vi "init_img_processing_vars.vi"(7 "Count Buffer Size 1":i32=2000000) -> (8 "Image Processing Data":T1)   [LabVIEW 2023]
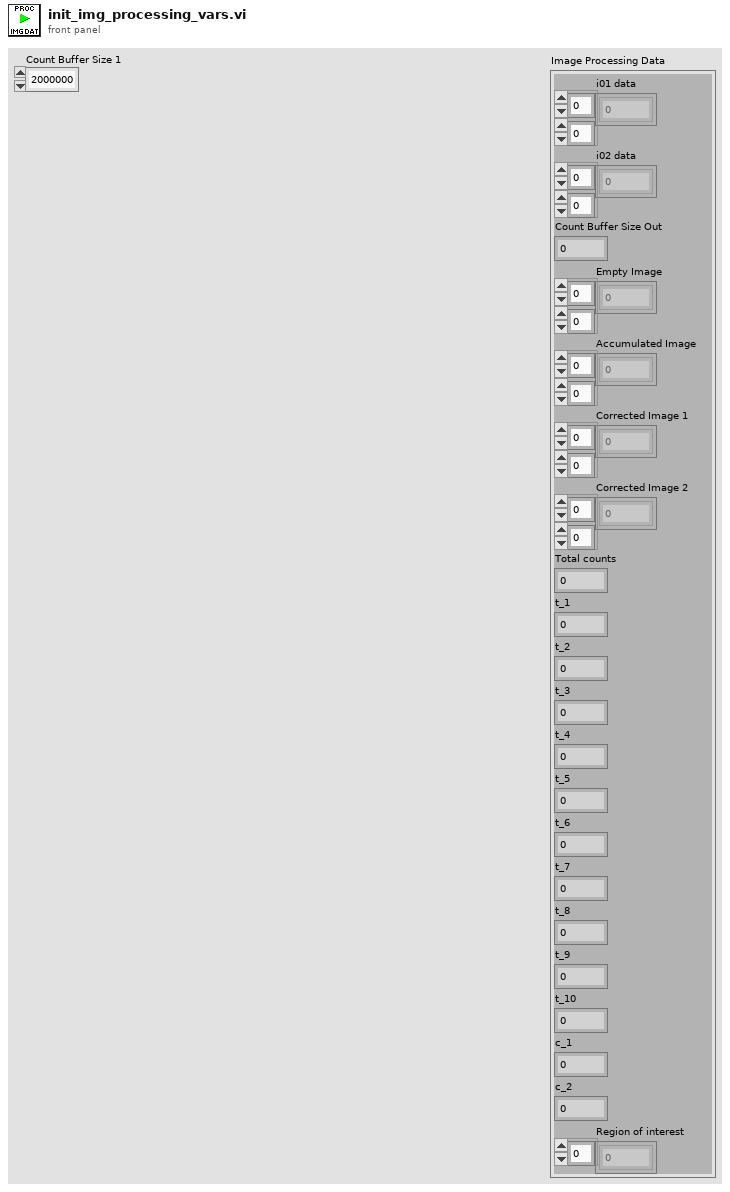
[diagram p1: front panel]
types:
  T1 = cluster{"i01 data":sgl[][], "i02 data":sgl[][], "Count Buffer Size Out":i32, "Empty Image":i16[][], "Accumulated Image":i16[][], "Corrected Image 1":i16[][], "Corrected Image 2":i16[][], "Total counts":i32, "t_1":i32, "t_2":i32, "t_3":i32, "t_4":i32, "t_5":i32, "t_6":i32, "t_7":i32, "t_8":i32, "t_9":i32, "t_10":i32, "c_1":i32, "c_2":i32, "Region of interest":i32[]}
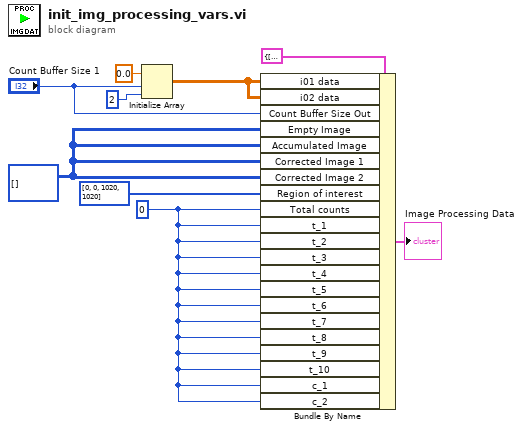
[diagram p0: block diagram]
diagram:
  w4 = i16[][] []
  w2 = 0
  n1 = Initialize Array(sgl 0.0 ("element"), "Count Buffer Size 1", 2 ("dimension size")) -> (w6:sgl[][])
  n2 = Bundle By Name(cluster=T1 {"i01 data"=[], "i02 data"=[], "Count Buffer Size Out"=2000000, "Empty Image"=[], "Accumulated Image"=[], "Corrected Image 1"=[], "Corrected Image 2"=[], "Total counts"=0, "t_1"=0, "t_2"=0, "t_3"=0, "t_4"=0, "t_5"=0, "t_6"=0, "t_7"=0, "t_8"=0, "t_9"=0, "t_10"=0, "c_1"=0, "c_2"=0, "Region of interest"=[0, 0, 1020, 1020]}, "i01 data"=w6, "i02 data"=w6, "Count Buffer Size Out"="Count Buffer Size 1", "Empty Image"=w4, "Accumulated Image"=w4, "Corrected Image 1"=w4, "Corrected Image 2"=w4, "Region of interest"=i32[] [0, 0, 1020, 1020], "Total counts"=w2, "t_1"=w2, "t_2"=w2, "t_3"=w2, "t_4"=w2, "t_5"=w2, "t_6"=w2, "t_7"=w2, "t_8"=w2, "t_9"=w2, "t_10"=w2, "c_1"=w2, "c_2"=w2) -> (→"Image Processing Data":T1)
